vi "Sleep Mano Menu.vi"(8 "error in":errorcluster, 11 "Data Cluster In":T1={"Selected File"=path "", "Full Text File"=[], "Data Array"=[], "Times Array"=[], "Sensor Array"=[], "Subset Array"=[], "Smoothness Values"=[], "Sensor Select 1"=refnum, "Sensor Select 2"=refnum, "Sensor Select 3"=refnum, "Sensor Select 4"=refnum, "Start Times"=[], "End Times"=[], "Cursor List"=[{"Name"="Event Marker          ", "Color"=16777200, "Style"=0, "Point Style"=0, "Name Visible"=FALSE, "Allow Drag"=FALSE, "Cursor Mode"=0, "Plot"=0, "Index"=0, "Position"={"X"=4.0, "Y"=1.0}, "X Scale"=0, "Y Scale"=0, "Watch Plots"=[], "Watch All Plots"=FALSE, "Plot Area"=0, "Label Offset"={"X"=-50.0, "Y"=150.0}}, {"Name"="Upper Sensor", "Color"=13816500, "Style"=6, "Point Style"=0, "Name Visible"=FALSE, "Allow Drag"=FALSE, "Cursor Mode"=0, "Plot"=0, "Index"=0, "Position"={"X"=-1.0, "Y"=5.0}, "X Scale"=0, "Y Scale"=0, "Watch Plots"=[], "Watch All Plots"=FALSE, "Plot Area"=0, "Label Offset"={"X"=0.0, "Y"=0.0}}, {"Name"="Lower Sensor", "Color"=13816500, "Style"=6, "Point Style"=0, "Name Visible"=FALSE, "Allow Drag"=FALSE, "Cursor Mode"=0, "Plot"=0, "Index"=0, "Position"={"X"=-1.0, "Y"=30.0}, "X Scale"=0, "Y Scale"=0, "Watch Plots"=[], "Watch All Plots"=FALSE, "Plot Area"=0, "Label Offset"={"X"=0.0, "Y"=0.0}}], "Listbox 1"=refnum, "Listbox 2"=refnum, "Listbox 3"=refnum, "Listbox 4"=refnum, "Labels"=["Why", "is", "this", "still", "not", "built", "into", "Labview?", "This", "is", "shameful."], "Event Array"=[], "Event Names"=[], "Event Times"=[], "Save Plot Button"=refnum, "Sensor Plot Refs"=[], "Selected Event (Title)"="", "Upper Cursor"=0.0, "Lower Cursor"=0.0, "Z Max"=0.0, "Z Min"=0.0}) -> (0 "error out":errorcluster, 3 "Data Cluster Out":T1={"Selected File"=path "", "Full Text File"=[], "Data Array"=[], "Times Array"=[], "Sensor Array"=[], "Subset Array"=[], "Smoothness Values"=[], "Sensor Select 1"=refnum, "Sensor Select 2"=refnum, "Sensor Select 3"=refnum, "Sensor Select 4"=refnum, "Start Times"=[], "End Times"=[], "Cursor List"=[{"Name"="Event Marker          ", "Color"=16777200, "Style"=0, "Point Style"=0, "Name Visible"=FALSE, "Allow Drag"=FALSE, "Cursor Mode"=0, "Plot"=0, "Index"=0, "Position"={"X"=4.0, "Y"=1.0}, "X Scale"=0, "Y Scale"=0, "Watch Plots"=[], "Watch All Plots"=FALSE, "Plot Area"=0, "Label Offset"={"X"=-50.0, "Y"=150.0}}, {"Name"="Upper Sensor", "Color"=13816500, "Style"=6, "Point Style"=0, "Name Visible"=FALSE, "Allow Drag"=FALSE, "Cursor Mode"=0, "Plot"=0, "Index"=0, "Position"={"X"=-1.0, "Y"=5.0}, "X Scale"=0, "Y Scale"=0, "Watch Plots"=[], "Watch All Plots"=FALSE, "Plot Area"=0, "Label Offset"={"X"=0.0, "Y"=0.0}}, {"Name"="Lower Sensor", "Color"=13816500, "Style"=6, "Point Style"=0, "Name Visible"=FALSE, "Allow Drag"=FALSE, "Cursor Mode"=0, "Plot"=0, "Index"=0, "Position"={"X"=-1.0, "Y"=30.0}, "X Scale"=0, "Y Scale"=0, "Watch Plots"=[], "Watch All Plots"=FALSE, "Plot Area"=0, "Label Offset"={"X"=0.0, "Y"=0.0}}], "Listbox 1"=refnum, "Listbox 2"=refnum, "Listbox 3"=refnum, "Listbox 4"=refnum, "Labels"=["Why", "is", "this", "still", "not", "built", "into", "Labview?", "This", "is", "shameful."], "Event Array"=[], "Event Names"=[], "Event Times"=[], "Save Plot Button"=refnum, "Sensor Plot Refs"=[], "Selected Event (Title)"="", "Upper Cursor"=0.0, "Lower Cursor"=0.0, "Z Max"=0.0, "Z Min"=0.0})   [LabVIEW 2020]
uses:
  Controls/Selector Cases.ctl
  Controls/DataCluster.ctl
  <vilib>/Utility/miscctls.llb/LVCursorListTypeDef.ctl
panel:
  in  "Starting State":T3
  out "Segment Select":dbl[][](graph)
  in  "Event Name":u16(ring) items=["2cc1", "2cc2", "2cc3", "2cc4", "2cc5", "2cc6", "2cc7", "2cc8", "2cc9", "2cc10", "10cc1", "10cc2", "10cc3", "10cc5", "10cc6", "10cc7", "10cc8", "10cc9", "10cc10", "self1", "self2", "self3", "self4", "self5", "self6", "self7", "5cc water1", "5cc water2", "5cc water3", "5cc lemon1", "5cc lemon2", "5cc lemon3", "5cc water4", "5cc water5", "5cc water6", "5cc lemon4", "5cc lenon5", "5cc lemon6", "5cc water7", "5cc water8", "5cc water9"]
  in  "Home Button":bool
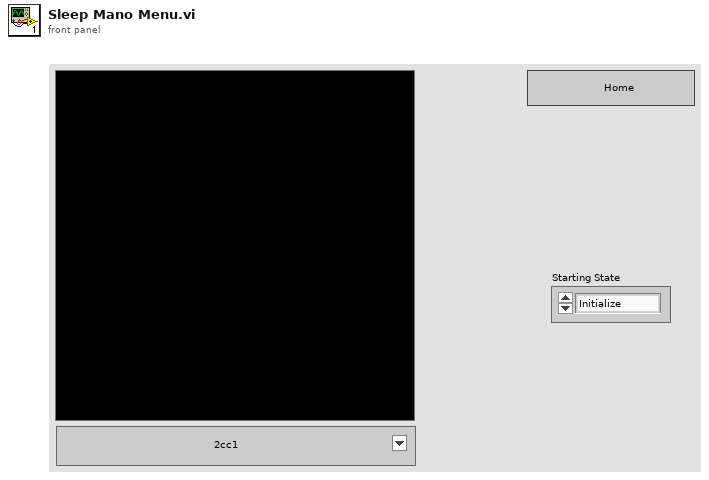
[diagram p1: front panel]
types:
  T1 = typedef "DataCluster.ctl" = cluster{"Selected File":path, "Full Text File":string[][], "Data Array":dbl[][], "Times Array":dbl[], "Sensor Array":dbl[], "Subset Array":dbl[][], "Smoothness Values":dbl[], "Sensor Select 1":refnum<vi>, "Sensor Select 2":refnum<vi>, "Sensor Select 3":refnum<vi>, "Sensor Select 4":refnum<vi>, "Start Times":dbl[], "End Times":dbl[], "Cursor List":T2, "Listbox 1":refnum<vi>, "Listbox 2":refnum<vi>, "Listbox 3":refnum<vi>, "Listbox 4":refnum<vi>, "Labels":string[], "Event Array":dbl[][], "Event Names":string[], "Event Times":dbl[], "Save Plot Button":refnum<vi>, "Sensor Plot Refs":refnum<vi>[], "Selected Event (Title)":string, "Upper Cursor":dbl, "Lower Cursor":dbl, "Z Max":dbl, "Z Min":dbl}
  T2 = typedef "LVCursorListTypeDef.ctl" = cluster{"Name":string, "Color":u32, "Style":u8, "Point Style":u8, "Name Visible":bool, "Allow Drag":bool, "Cursor Mode":u32, "Plot":i32, "Index":i32, "Position":cluster{"X":dbl, "Y":dbl}, "X Scale":u32, "Y Scale":u32, "Watch Plots":i32[], "Watch All Plots":bool, "Plot Area":i32, "Label Offset":cluster{"X":dbl, "Y":dbl}}[]
  T3 = typedef "Selector Cases.ctl" = enum16{"Initialize", "Wait", "Open", "Find Segment", "Update Sensor Plots", "Analyze", "Save", "Exit"}
  T4 = enum16{"None", "On Hover", "On Key Focus", "On Hover or Key Focus"}
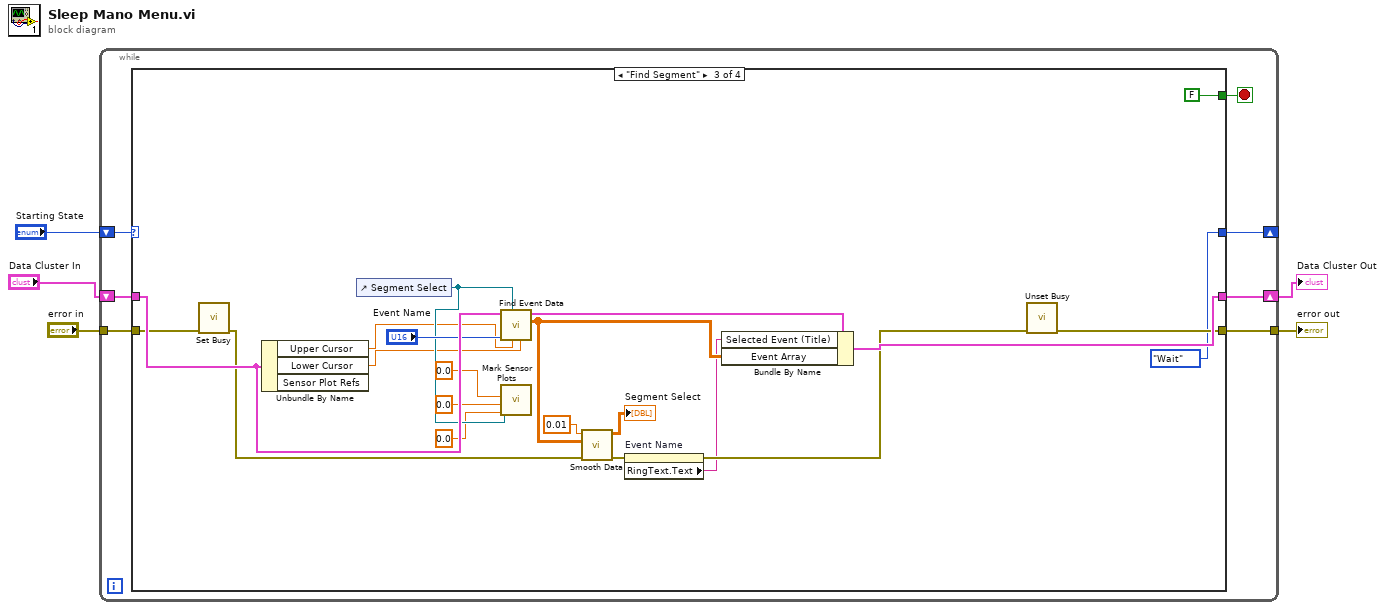
[diagram p0: block diagram]
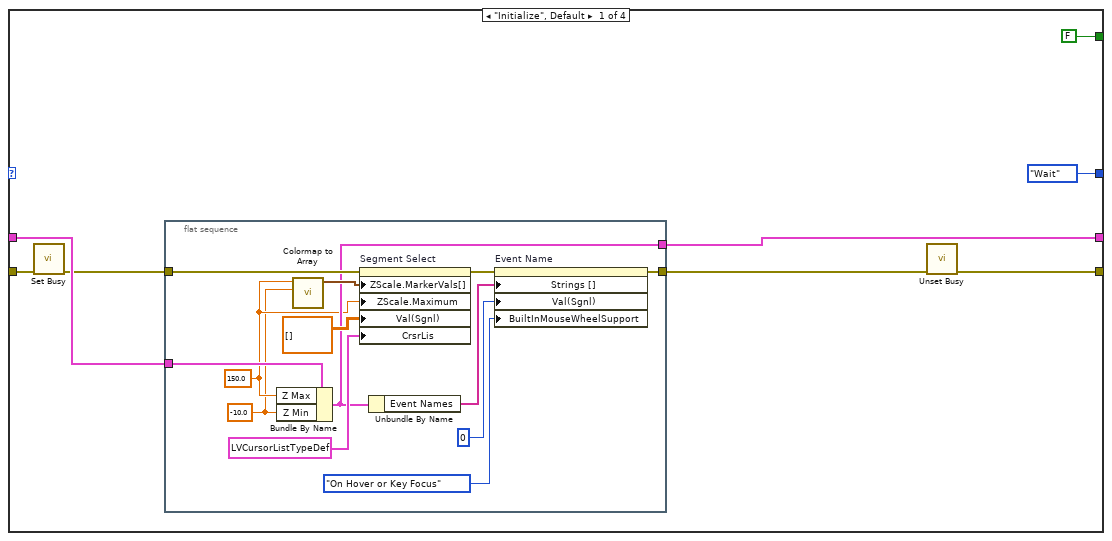
[diagram p2: hidden frame]
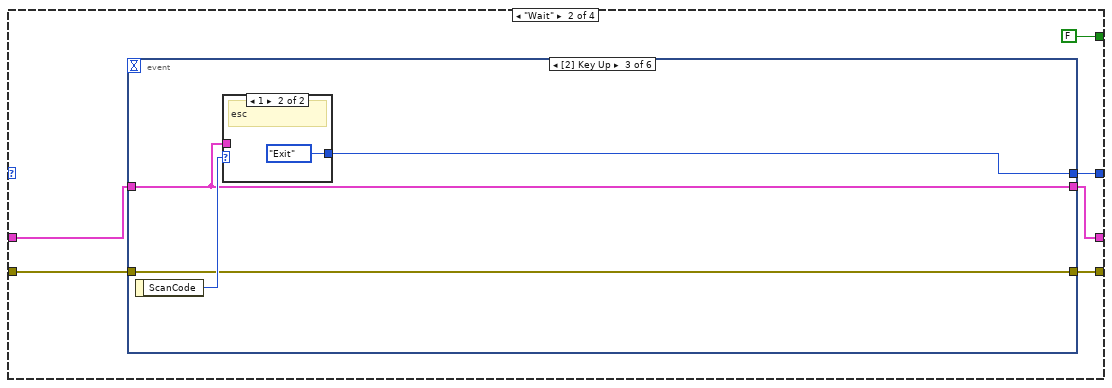
[diagram p3: hidden frame]
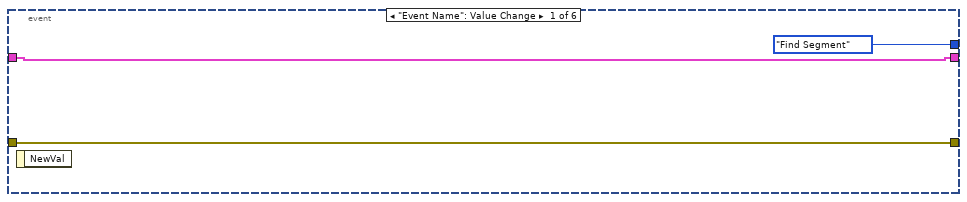
[diagram p4: hidden frame]
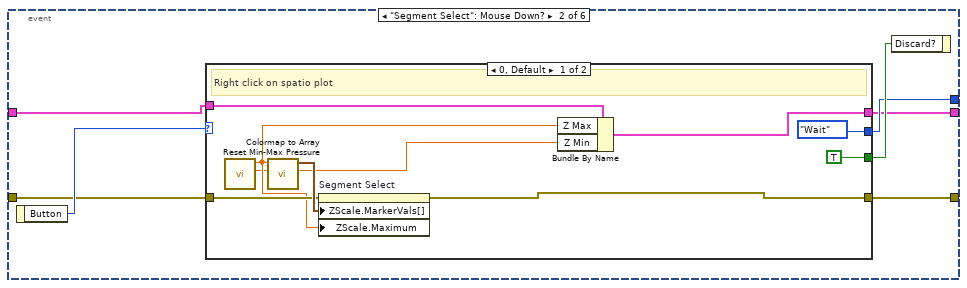
[diagram p5: hidden frame]
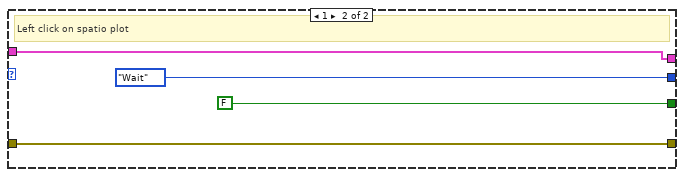
[diagram p6: hidden frame]
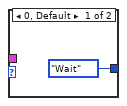
[diagram p7: hidden frame]
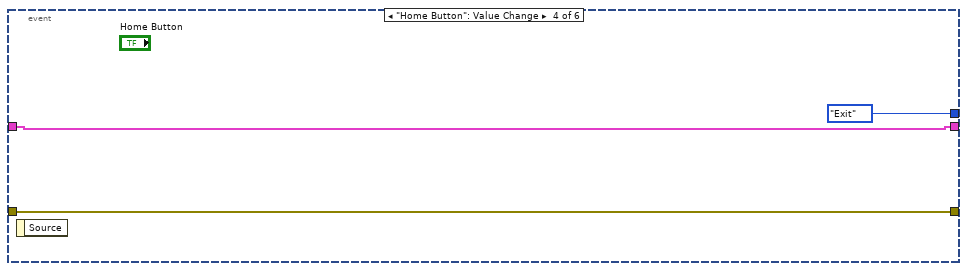
[diagram p8: hidden frame]
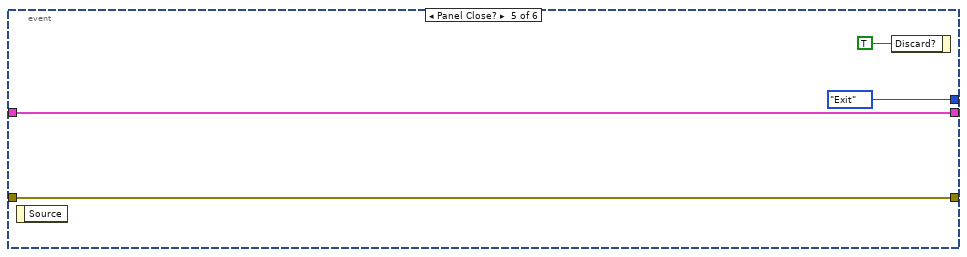
[diagram p9: hidden frame]
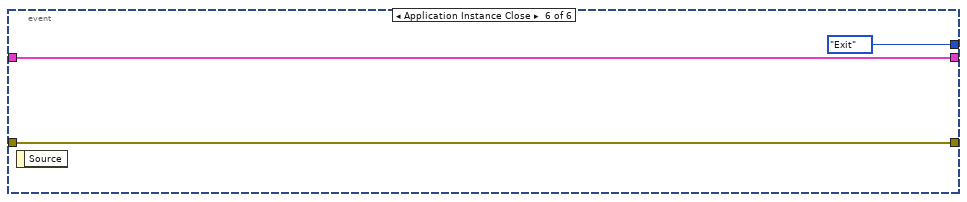
[diagram p10: hidden frame]
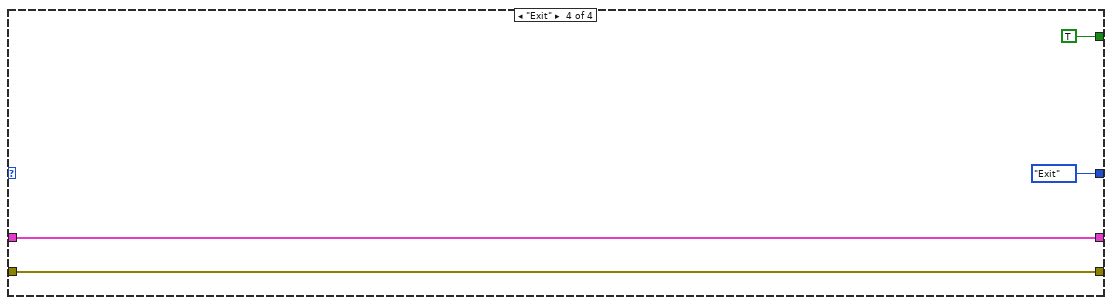
[diagram p11: hidden frame]
diagram:
  n1 = while {
    shift-right: [w10] -> _
    shift-left: "Starting State" -> [w12]
    shift-right: [w6] -> w1
    shift-left: "Data Cluster In" -> [w9]
    tunnel: "error in" -> [w8]
    tunnel: [w7] -> w4
    stop <- w11 stop-if-true
    n2 = case shown="\"Find Segment\"" w12 {
      tunnel: [FALSE FALSE FALSE TRUE] -> w11
      tunnel: [Selector_Cases."Wait" ("Starting State 2") w38 Selector_Cases."Wait" ("Starting State") Selector_Cases."Exit" ("Starting State")] -> w10
      tunnel: w9 -> [w19 w35 w97 w101]
      tunnel: [w14 w34 w98 w101] -> w6
      tunnel: w8 -> [w17 w37 w96 w102]
      tunnel: [w15 w36 w93 w102] -> w7
      frame "Initialize", Default {
        n3 = call <vilib>:"Set Busy.vi"("error in (no error)"=w17) -> ("error out"=w18:errorcluster)  [unwired: 9 in, 1 out]
        n4 = flat-sequence {
          tunnel: w19 -> [w24]
          tunnel: [w26] -> w14
          tunnel: w18 -> [w33]
          tunnel: [w32] -> w16
          frame #0 {
            w22 = -10.0 ("Min Pressure")
            w23 = 150.0 ("Max Pressure")
            n5 = Bundle By Name(cluster=w24, "Z Max"=w23, "Z Min"=w22) -> (w26:T1)
            n6 = call "Colormap to Array.vi"("Min Pressure"=w22, "Max Pressure"=w23) -> ("Z Scale.Marker Values[]"=w30:cluster{dbl, u32}[])  [unwired: 9 in]
            n7 = property on="Segment Select" class="IntGraph (strict)"(error in=w33, "ZScale.MarkerVals[]"=w30, "ZScale.Maximum"=w23, "Val(Sgnl)"=dbl[][] [] ("Value (Signaling)"), "CrsrLis"=T2 [{"Name"="Event Marker          ", "Color"=16777200, "Style"=0, "Point Style"=0, "Name Visible"=FALSE, "Allow Drag"=FALSE, "Cursor Mode"=0, "Plot"=0, "Index"=0, "Position"={"X"=4.0, "Y"=0.0}, "X Scale"=0, "Y Scale"=0, "Watch Plots"=[], "Watch All Plots"=FALSE, "Plot Area"=0, "Label Offset"={"X"=-50.0, "Y"=150.0}}, {"Name"="Upper Sensor", "Color"=13816500, "Style"=6, "Point Style"=0, "Name Visible"=FALSE, "Allow Drag"=FALSE, "Cursor Mode"=0, "Plot"=0, "Index"=0, "Position"={"X"=-1.0, "Y"=5.0}, "X Scale"=0, "Y Scale"=0, "Watch Plots"=[], "Watch All Plots"=FALSE, "Plot Area"=0, "Label Offset"={"X"=0.0, "Y"=0.0}}, {"Name"="Lower Sensor", "Color"=13816500, "Style"=6, "Point Style"=0, "Name Visible"=FALSE, "Allow Drag"=FALSE, "Cursor Mode"=0, "Plot"=0, "Index"=0, "Position"={"X"=-1.0, "Y"=30.0}, "X Scale"=0, "Y Scale"=0, "Watch Plots"=[], "Watch All Plots"=FALSE, "Plot Area"=0, "Label Offset"={"X"=0.0, "Y"=0.0}}] ("Cursor List")) -> (error out=w21:errorcluster)  [unwired: 1 in, 1 out]
            n8 = Unbundle By Name(w26) -> ("Event Names"=w25:string[])
            n9 = property on="Event Name" class="Ring (strict)"(error in=w21, "Strings []"=w25, "Val(Sgnl)"=u16 0 ("Value (Signaling)"), "BuiltInMouseWheelSupport"=T4."On Hover or Key Focus" ("Built-In Mouse Wheel Support")) -> (error out=w32:errorcluster)  [unwired: 1 in, 1 out]
          }
        }
        n10 = call <vilib>:"Unset Busy.vi"("error in (no error)"=w16) -> ("error out"=w15:errorcluster)  [unwired: 10 in]
      }
      frame "Wait" {
        n11 = event shown="[2] Key Up" {
          selector: _ -> [_ _ _ _ _ _]
          dyn-events: _ -> [_ _ _ _ _ _]
          timeout: _ -> [_ _ _ _ _ _]
          tunnel: [Selector_Cases."Find Segment" ("Starting State") w45 w66 Selector_Cases."Exit" ("Starting State") Selector_Cases."Exit" ("Starting State") Selector_Cases."Exit" ("Starting State")] -> w38
          tunnel: w35 -> [w41 w44 w63 w71 w74 w77]
          tunnel: w37 -> [w42 w47 w64 w70 w75 w78]
          tunnel: [w42 w48 w64 w70 w75 w78] -> w36
          tunnel: [w41 w43 w63 w71 w74 w77] -> w34
          event "Event Name": Value Change {
            n12 = event-data() -> ()  [unwired: 1 in, 1 out]
          }
          event "Segment Select": Mouse Down? {
            n13 = event-data() -> ("Button"=w49:u16)  [unwired: 1 in]
            n14 = case shown="0, Default" w49 {
              tunnel: [w50 w62] -> w48
              tunnel: w47 -> [w56 w62]
              tunnel: [TRUE FALSE] -> w46
              tunnel: [Selector_Cases."Wait" ("Starting State") Selector_Cases."Wait" ("Starting State")] -> w45
              tunnel: w44 -> [w55 w60]
              tunnel: [w54 w60] -> w43
              frame 0, Default {
                # "Right click on spatio plot"
                n15 = call "Reset Min-Max Pressure.vi"() -> ("Min Pressure Out"=w52:dbl, "Max Pressure Out"=w53:dbl)  [unwired: 10 in]
                n16 = call "Colormap to Array.vi"("Min Pressure"=w52, "Max Pressure"=w53) -> ("Z Scale.Marker Values[]"=w57:cluster{dbl, u32}[])  [unwired: 9 in]
                n17 = property on="Segment Select" class="IntGraph (strict)"(error in=w56, "ZScale.MarkerVals[]"=w57, "ZScale.Maximum"=w53) -> (error out=w50:errorcluster)  [unwired: 1 in, 1 out]
                n18 = Bundle By Name(cluster=w55, "Z Max"=w53, "Z Min"=w52) -> (w54:T1)
              }
              frame 1 {
                # "Left click on spatio plot"
              }
            }
            n19 = event-data("Discard?"=w46) -> ()  [unwired: 1 in, 1 out]
          }
          event Key Up {
            n20 = event-data() -> ("ScanCode"=w65:i16)  [unwired: 1 in]
            n21 = case shown="1" w65 {
              tunnel: [Selector_Cases."Wait" ("Starting State") Selector_Cases."Exit" ("Starting State")] -> w66
              tunnel: w63 -> [_ _]
              frame 0, Default {
              }
              frame 1 {
                # "esc"
              }
            }
          }
          event "Home Button": Value Change {
            n22 = event-data() -> ()  [unwired: 1 in, 1 out]
          }
          event Panel Close? {
            n23 = event-data() -> ()  [unwired: 1 in, 1 out]
            n24 = event-data("Discard?"=TRUE) -> ()  [unwired: 1 in, 1 out]
          }
          event Application Instance Close {
            n25 = event-data() -> ()  [unwired: 1 in, 1 out]
          }
        }
      }
      frame "Find Segment" {
        n26 = call <vilib>:"Set Busy.vi"("error in (no error)"=w96) -> ("error out"=w95:errorcluster)  [unwired: 9 in, 1 out]
        n27 = Unbundle By Name(w97) -> ("Upper Cursor"=w81:dbl, "Lower Cursor"=w80:dbl)  [unwired: 1 out]
        n28 = control-ref of="Segment Select"() -> (w86:refnum<vi>)
        n29 = call "Find Event Data.vi"("Lower Sensor"=w80, "Upper Sensor"=w81, "Intensity Plot Ref"=w86, "Event Name"="Event Name", "Data Cluster In"=w97) -> ("Event Data Array"=w88:dbl[][], "output cluster"=w90:T1)  [unwired: 5 in]
        n30 = call "Mark Sensor Plots.vi"("Segment Select Ref"=w86, "Segement Start"=0.0, "End"=0.0, "Start"=0.0) -> ()  [unwired: 7 in]
        n31 = call "Smooth Data.vi"("error in (no error)"=w95, "Data Array"=w88, "dt"=0.01) -> ("error out"=w82:errorcluster, "Resampled Array"=→"Segment Select":dbl[][])  [unwired: 7 in]
        n32 = property on="Event Name" class="Ring (strict)"(error in=w82) -> (error out=w94:errorcluster, "RingText.Text"=w79:string)  [unwired: 1 in, 1 out]
        n33 = Bundle By Name(cluster=w90, "Selected Event (Title)"=w79, "Event Array"=w88) -> (w98:T1)
        n34 = call <vilib>:"Unset Busy.vi"("error in (no error)"=w94) -> ("error out"=w93:errorcluster)  [unwired: 10 in]
      }
      frame "Exit" {
      }
    }
  }
  "error out" <- w4
  "Data Cluster Out" <- w1
